vi "Plugin Template.vi"() -> ()   [LabVIEW 2021]
uses:
  <vilib>/Plug-In SDKs/InstrumentStudio SDK/InstrumentStudioPluginSDK.lvlibp/Plugin Session.lvclass
  <vilib>/Plug-In SDKs/InstrumentStudio SDK/InstrumentStudioPluginSDK.lvlibp/Plugin Events Enum.ctl
  <vilib>/Plug-In SDKs/InstrumentStudio SDK/InstrumentStudioPluginSDK.lvlibp
panel:
  in  "Session Id":u64
types:
  T1 = typedef "InstrumentStudioPluginSDK.lvlibp/Plugin Events Enum.ctl" = enum16{"Shutdown", "Project Saved", "Stop All Outputs"}
  T2 = typedef "InstrumentStudioPluginSDK.lvlibp/Event Registration Refnum.ctl" = refnum<event-registration>
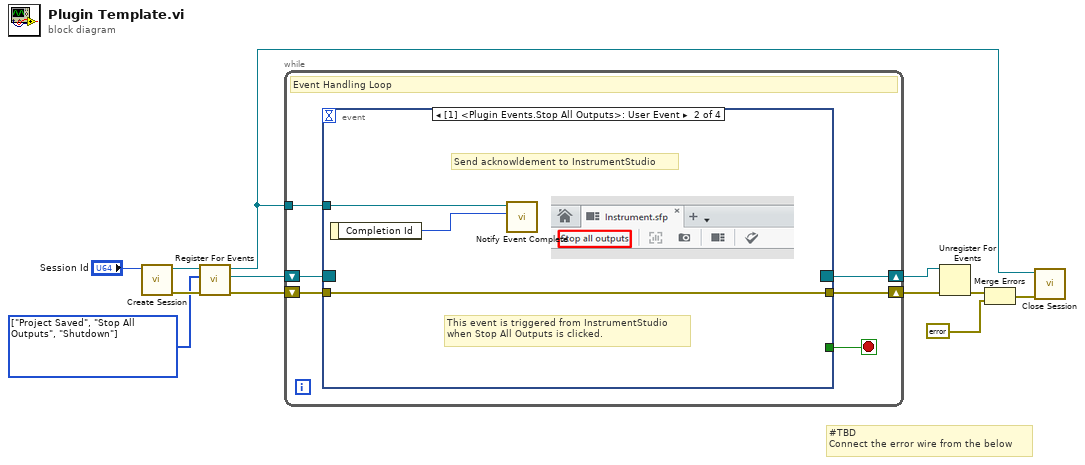
[diagram p0: block diagram]
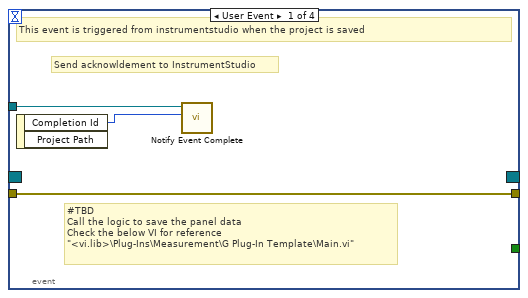
[diagram p2: hidden frame]
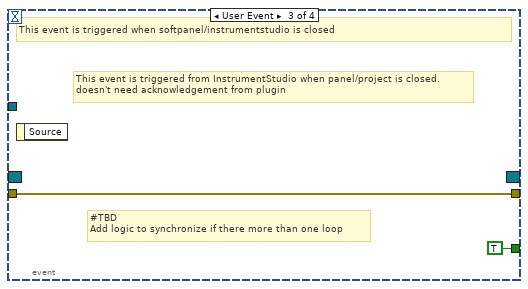
[diagram p3: hidden frame]
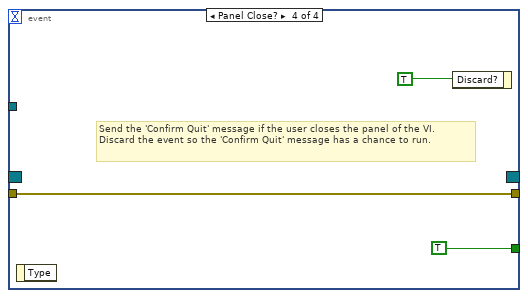
[diagram p4: hidden frame]
diagram:
  w9 = T1[] [enum."Project Saved", enum."Stop All Outputs", enum."Shutdown"] items=["Shutdown", "Project Saved", "Stop All Outputs"] ("Events To Register")
  # "#TBD\nConnect the error wire from the below"
  n1 = call <vilib>:"Create Session.vi"("Session Id"="Session Id") -> ("error out"=w11:errorcluster, "Session out"=w10:refnum<class "Plugin Session.lvclass">)  [unwired: 6 in, 3 out]
  n2 = call <vilib>:"Register For Events.vi"("error in (no error)"=w11, "Events To Register"=w9, "Session in"=w10) -> ("error out"=w8:errorcluster, "Event Refnum"=w5:T2, "Session out"=w3:refnum<class "Plugin Session.lvclass">)  [unwired: 6 in]
  n3 = while {
    shift-right: [w17] -> w6
    shift-left: w5 -> [w18]
    tunnel: w3 -> [w15]
    shift-right: [w13] -> w7
    shift-left: w8 -> [w14]
    stop <- w16 stop-if-true
    # "Event Handling Loop"
    n4 = event shown="[1] <Plugin Events.Stop All Outputs>: User Event" {
      selector: w18 -> [_ _ _ _]
      dyn-events: [_ _ _ _] -> w17
      timeout: _ -> [_ _ _ _]
      tunnel: [_ _ TRUE ("Discard?") TRUE ("Discard?")] -> w16
      tunnel: w15 -> [w21 w24 _ _]
      tunnel: w14 -> [w19 w22 w25 w27]
      tunnel: [w19 w22 w25 w27] -> w13
      event User Event {
        # "#TBD\nCall the logic to save the panel data\nCheck the below VI for reference\n\"<vi.lib>\\Plug-Ins\\Measurement\\G Plug-In Template\\Main.vi\""
        # "Send acknowldement to InstrumentStudio"
        # "This event is triggered from instrumentstudio when the project is saved"
        n5 = event-data() -> ("Completion Id"=w20:i64)  [unwired: 1 in, 1 out]
        n6 = call <vilib>:"Notify Event Complete.vi"("Completion Id"=w20, "Session in"=w21) -> ()  [unwired: 8 in, 2 out]
      }
      event User Event {
        # "This event is triggered from InstrumentStudio \nwhen Stop All Outputs is clicked."
        # "Send acknowldement to InstrumentStudio"
        n7 = event-data() -> ("Completion Id"=w23:i64)  [unwired: 1 in]
        n8 = call <vilib>:"Notify Event Complete.vi"("Completion Id"=w23, "Session in"=w24) -> ()  [unwired: 8 in, 2 out]
      }
      event User Event {
        # "#TBD\nAdd logic to synchronize if there more than one loop"
        # "This event is triggered from InstrumentStudio when panel/project is closed.\ndoesn't need acknowledgement from plugin"
        # "This event is triggered when softpanel/instrumentstudio is closed"
        n9 = event-data() -> ()  [unwired: 1 in, 1 out]
      }
      event Panel Close? {
        # "Send the 'Confirm Quit' message if the user closes the panel of the VI. Discard the event so the 'Confirm Quit' message has a chance to run."
        n10 = event-data() -> ()  [unwired: 1 in, 1 out]
        n11 = event-data("Discard?"=TRUE) -> ()  [unwired: 1 in, 1 out]
      }
    }
  }
  n12 = Unregister For Events(event registration refnum=w6, error in=w7) -> (error out=w4:errorcluster)
  n13 = Merge Errors(w4, errorcluster {"status"=FALSE, "code"=0, "source"=""} ("error in")) -> (w2:errorcluster)
  n14 = call <vilib>:"Close Session.vi"("error in (no error)"=w2, "Session in"=w3) -> ()  [unwired: 9 in, 1 out]
